vi "Test.vi"() -> ()   [LabVIEW 2017]
uses:
  <userlib>/_NEVSTOP/JKI State Machine ++/_Support/_JKISMQFGV.vi
  <userlib>/_NEVSTOP/JKI State Machine ++/JKI-State-Machine-Plus.lvlib
panel:
  out "State History":string
  in  "Name(\"\" to use uuid)":string="Event JKISM"
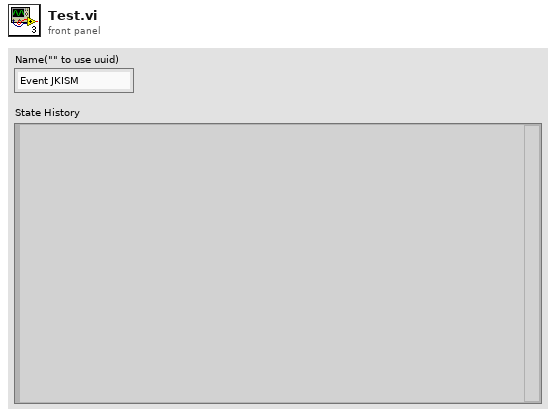
[diagram p1: front panel]
types:
  T1 = enum32{"Invalid", "Standard", "Closed", "Hidden", "Minimized", "Maximized"}
  T2 = enum32{"invalid app kind", "Development System", "Run Time System", "Student Edition", "Embedded LabVIEW", "Evaluation", "Custom"}
  T3 = cluster{"Core":cluster{"Current VI Reference":refnum<vi>, "Close Panel on Exit?":bool}, "Your Boolean data":bool, "Your string data":string}
  T4 = cluster{"Current VI Reference":refnum<vi>, "Close Panel on Exit?":bool}
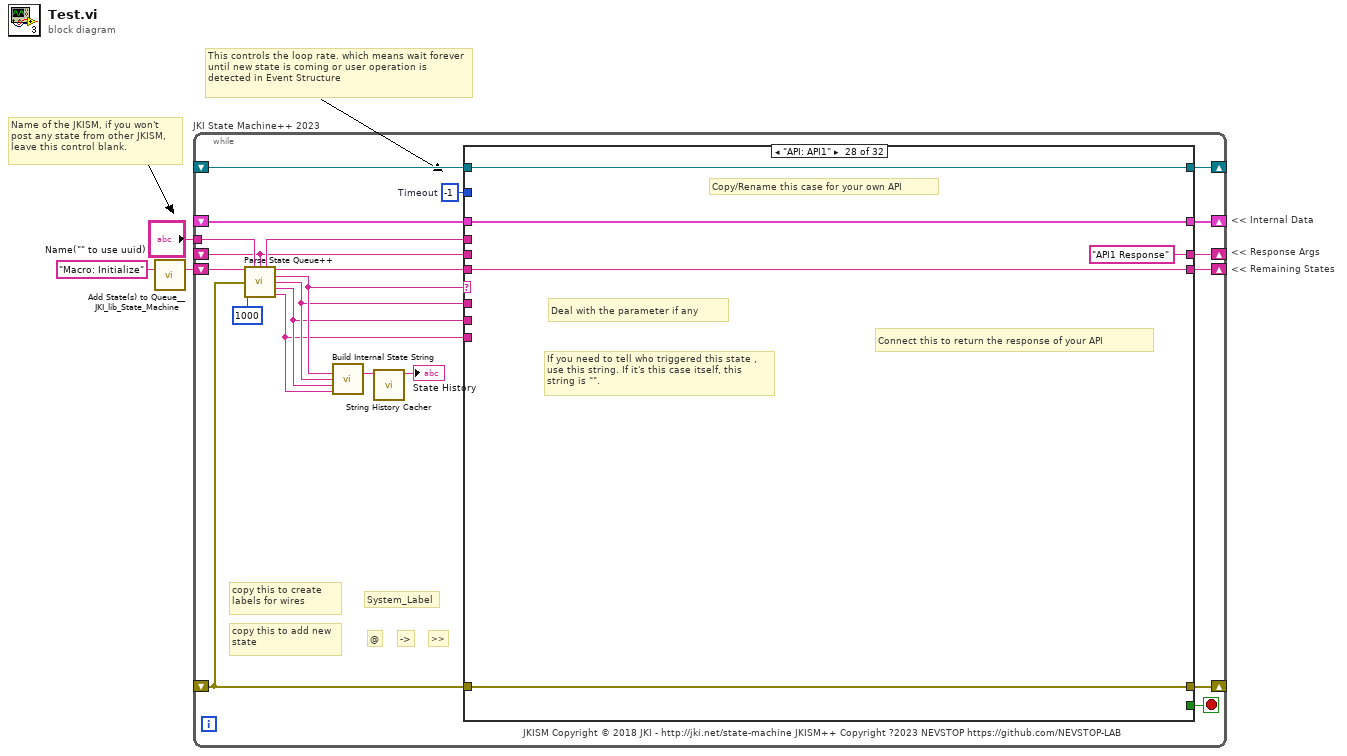
[diagram p0: block diagram]
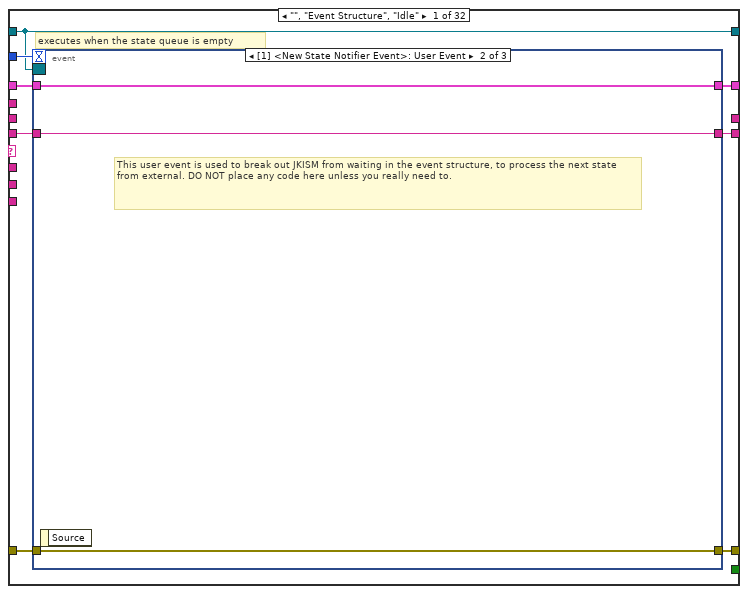
[diagram p2: hidden frame]
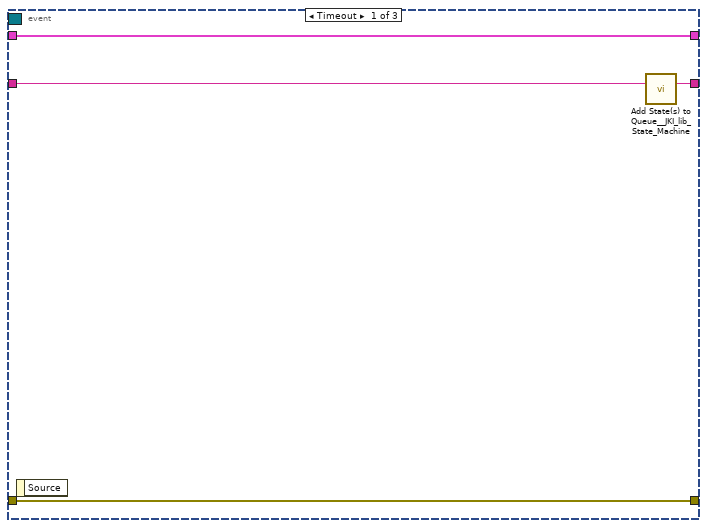
[diagram p3: hidden frame]
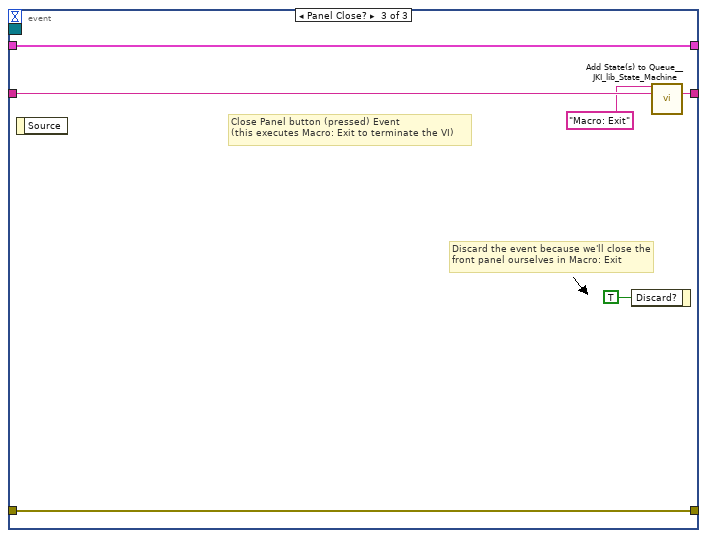
[diagram p4: hidden frame]
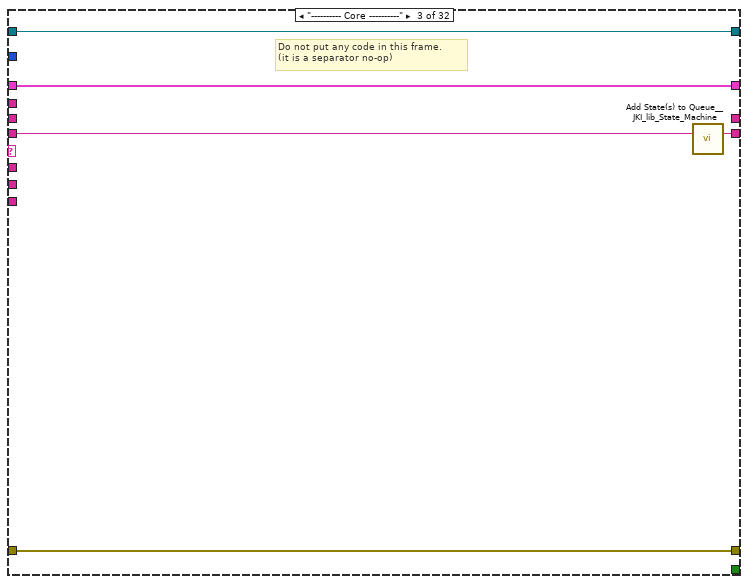
[diagram p6: hidden frame]
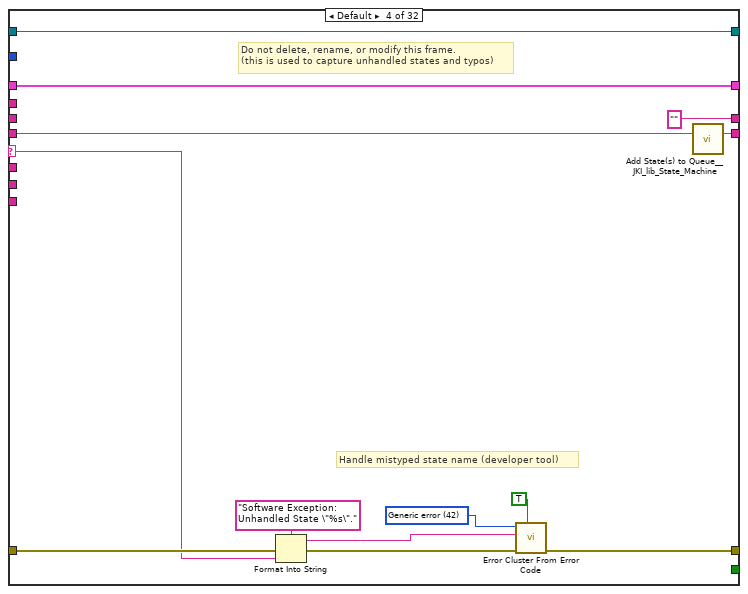
[diagram p7: hidden frame]
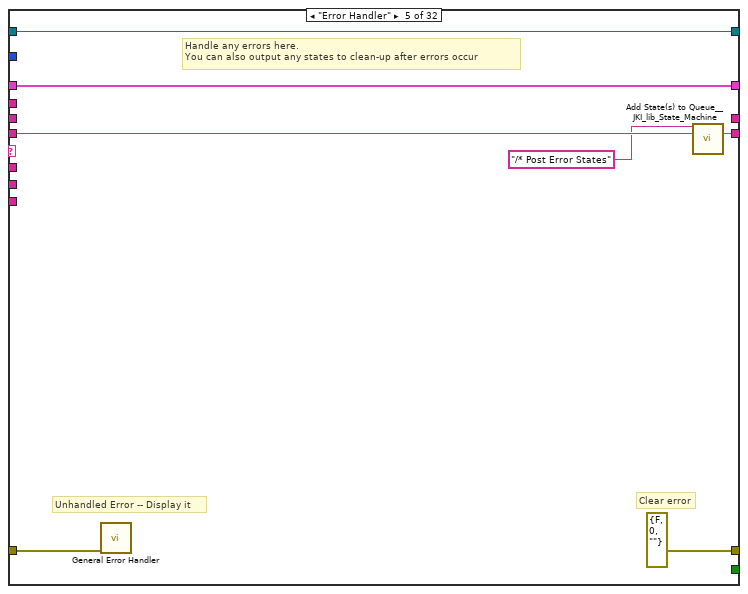
[diagram p8: hidden frame]
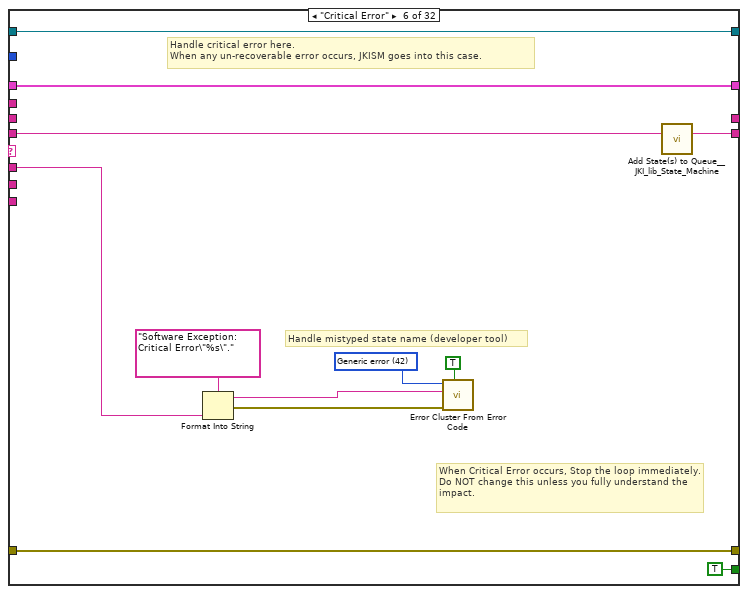
[diagram p9: hidden frame]
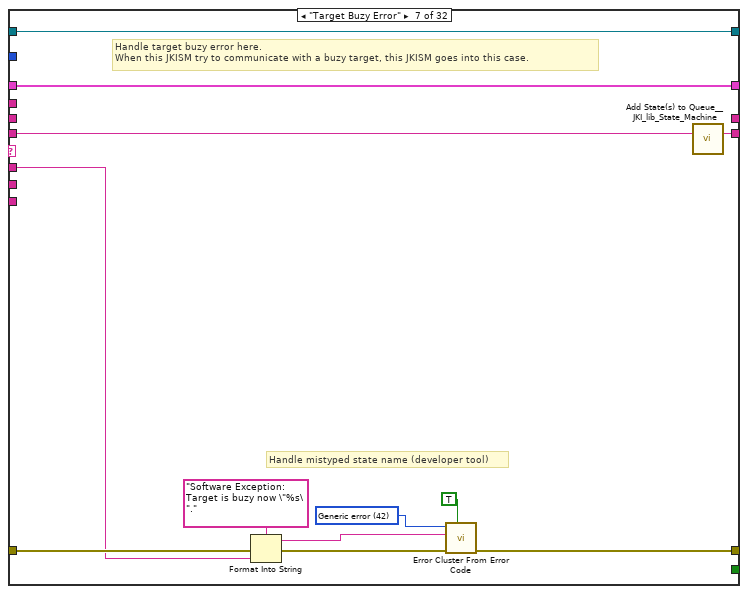
[diagram p10: hidden frame]
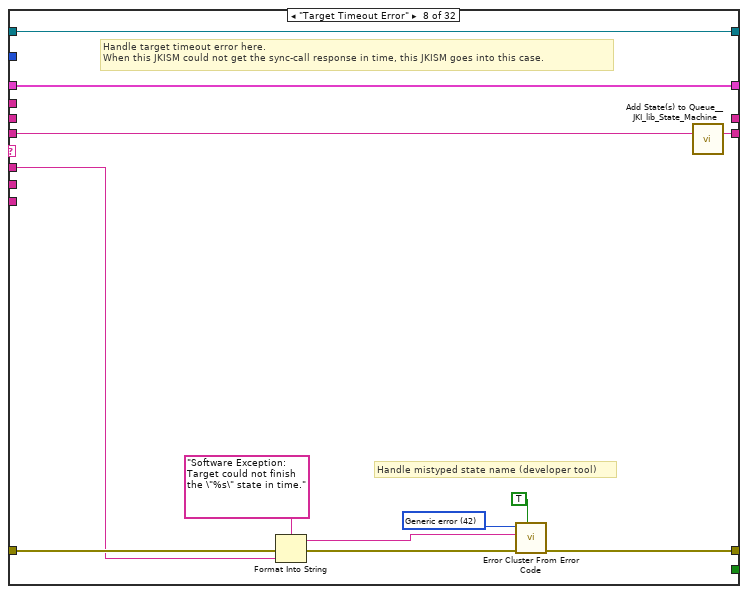
[diagram p11: hidden frame]
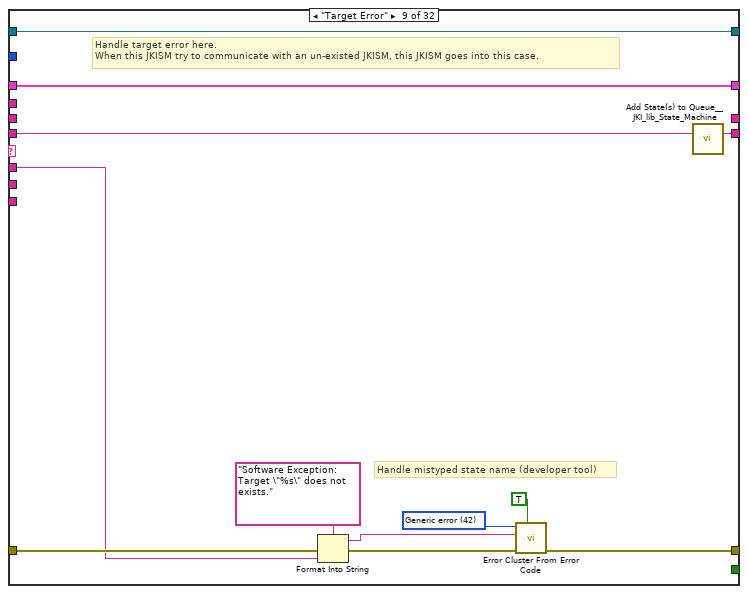
[diagram p12: hidden frame]
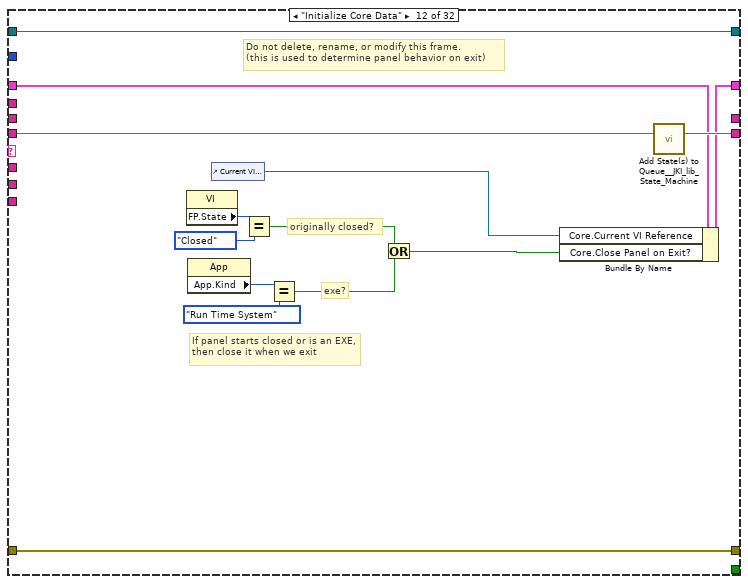
[diagram p15: hidden frame]
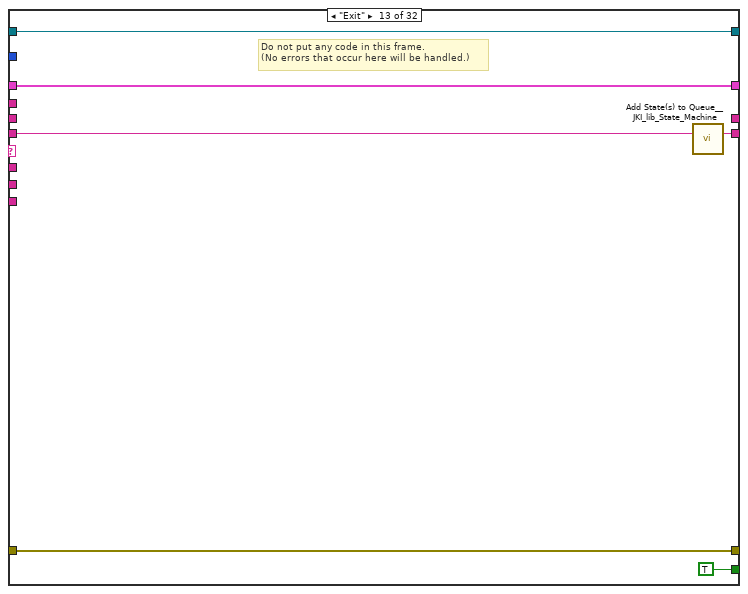
[diagram p16: hidden frame]
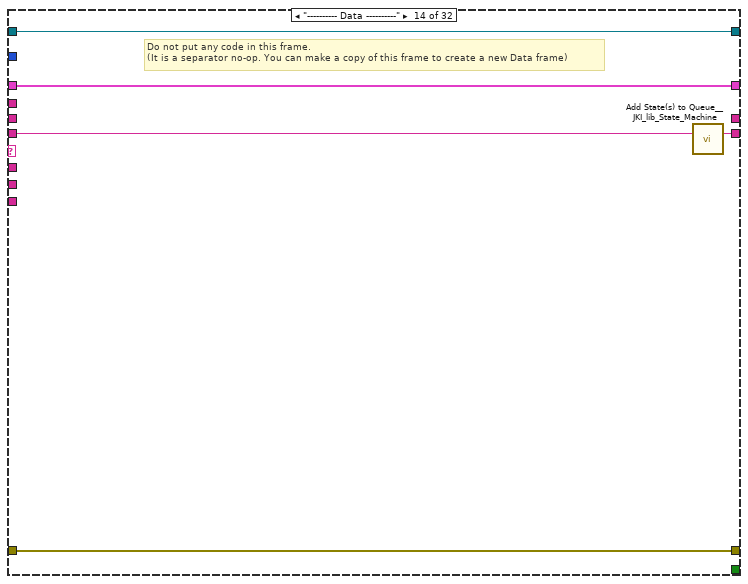
[diagram p17: hidden frame]
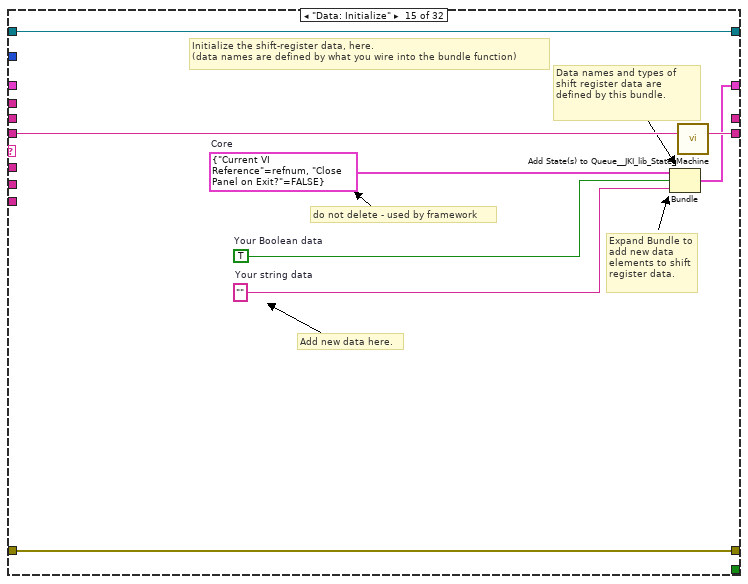
[diagram p18: hidden frame]
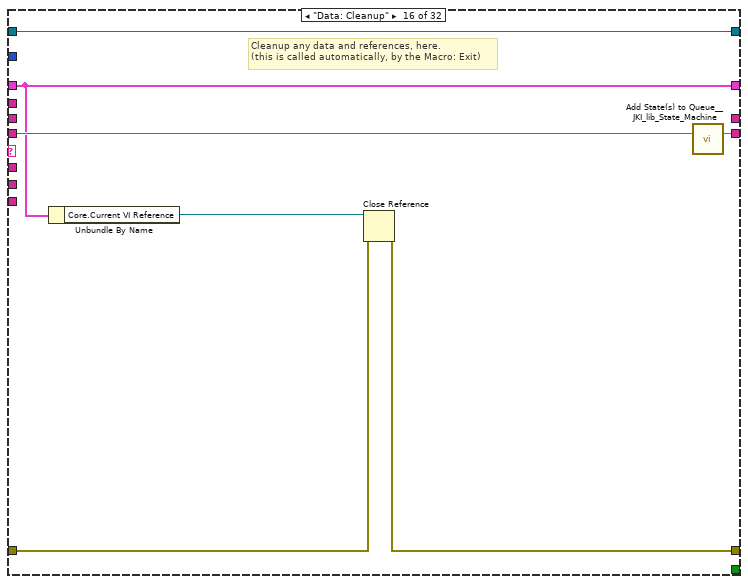
[diagram p19: hidden frame]
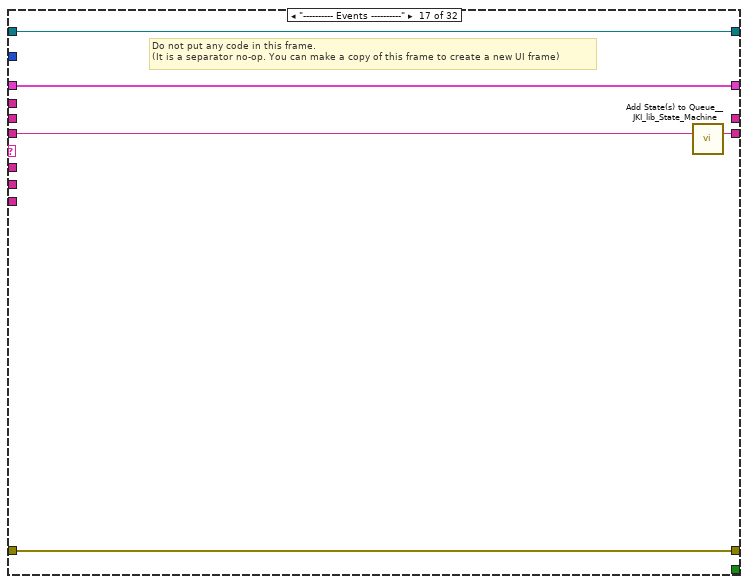
[diagram p20: hidden frame]
diagram:
  # "<< Internal Data"
  # "<< Response Args"
  # "<< Remaining States"
  # "Name of the JKISM, if you won't post any state from other JKISM,  leave this control blank."
  # "This controls the loop rate. which means wait forever until new state is coming or user operation is detected in Event Structure"
  n1 = call <vilib>:"Add State(s) to Queue__JKI_lib_State_Machine.vi"("State(s) in (\"\")"="Macro: Initialize") -> ("States Out"=w1:string)  [unwired: 14 in]
  n2 = while "JKI State Machine++ 2023" {
    shift-right: [w20] -> _
    shift-left: _ -> [w19]
    shift-right: [w23] -> _
    shift-left: _ -> [w17]
    shift-right: [w22] -> _
    shift-left: w1 -> [w24]
    tunnel: "Name(\"\" to use uuid)" -> [w12]
    shift-right: [w15] -> _
    shift-left: _ -> [w4]
    shift-right: [w14] -> _
    shift-left: _ -> [w13]
    stop <- w21 stop-if-true
    w18 = -1  # Timeout
    # "JKISM Copyright © 2018 JKI - http://jki.net/state-machine JKISM++ Copyright ?2023 NEVSTOP https://github.com/NEVSTOP-LAB"
    # "copy this to add new state"
    # ">>"
    # "->"
    # "@"
    # "copy this to create labels for wires"
    # "System_Label"
    n3 = call <userlib>:"Parse State Queue++.vi"("State Queue"=w24, "Name(\"\" to use uuid)"=w12, "Response Arguments"=w4, "Error In (no error)"=w17, "Response Timeout(5000ms)"=1000 ("Response Timeout(1000ms)")) -> ("Name Used"=w5:string, "Remaining States"=w25:string, "Current State"=w9:string, "Arguments"=w8:string, "Argument - State"=w7:string, "From Who"=w6:string)  [unwired: 5 in]
    n4 = call <userlib>:"Build Internal State String.vi"("State"=w9, "Arguments (\"\")"=w8, "Arg-State (\"\")"=w7, "Source (\"\")"=w6) -> ("State with Arguments"=w10:string)  [unwired: 11 in]
    n5 = call <userlib>:"String History Cacher.vi"("String"=w10) -> ("String Cache"=→"State History":string)  [unwired: 10 in]
    n6 = case shown="\"API: API1\"" w9 {
      selector: w9 -> [_ _ _ w58 _ _ _ _ _ _ _ _ _ _ _ _ _ _ _ _ _ _ _ _ _ _ _ _ _ _ _ _]
      tunnel: w25 -> [w33 w49 w55 w62 w75 w85 w88 w105 w117 w126 w130 w145 w151 w156 w164 w171 w176 w182 w186 w192 w197 w204 w216 w286 w292 w303 w306 w311 w317 w325 w331 w337]
      tunnel: w8 -> [_ _ _ _ _ w78 w90 w101 w113 _ _ _ _ _ _ _ _ _ _ _ _ w199 w210 _ _ _ _ _ w314 _ _ _]
      tunnel: w19 -> [w31 w48 w52 w60 w72 w86 w92 w103 w115 w125 w129 w138 w149 w153 _ w166 w173 w181 w185 w189 w195 w202 w212 w283 w289 w300 w305 w310 w316 w322 w328 w334]
      tunnel: [w30 w50 w53 w64 errorcluster {"status"=FALSE, "code"=0, "source"=""} ("error out") w87 w95 w107 w119 w127 w131 w142 w148 w154 w161 w167 w174 w177 w184 w190 w194 w200 w213 w284 w290 w301 w307 w312 w318 w323 w329 w335] -> w23
      tunnel: w17 -> [w29 w50 w53 w63 w71 w87 w94 w106 w118 w127 w131 w142 w148 w154 w161 w168 w174 _ w187 w190 w194 w201 w214 w284 w290 w301 w307 w312 w318 w323 w329 w335]
      tunnel: [w32 w49 w54 w61 w74 w84 w93 w104 w116 w126 w130 w144 w150 w155 w163 w170 w175 w182 w186 w191 w196 w203 w215 w285 w291 w302 w306 w311 w317 w324 w330 w336] -> w22
      tunnel: [_ _ _ _ _ TRUE _ _ _ _ _ _ TRUE _ _ _ _ _ _ _ _ _ _ _ _ _ _ _ _ _ _ _] -> w21
      tunnel: [w28 w48 w52 w60 w72 w86 w92 w103 w115 w125 w129 w143 w149 w153 w162 w166 w173 w181 w185 w189 w195 w202 w212 w283 w289 w300 w305 w310 w316 w322 w328 w334] -> w20
      tunnel: w18 -> [w27 _ _ _ _ _ _ _ _ _ _ _ _ _ _ _ _ _ _ _ _ _ _ _ _ _ _ _ _ _ _ _]
      tunnel: w6 -> [_ _ _ _ _ _ _ _ _ _ _ _ _ _ _ _ _ _ _ _ _ _ _ _ _ _ _ _ _ _ _ _]
      tunnel: w7 -> [_ _ _ _ _ _ _ _ _ _ _ _ _ _ _ _ _ _ _ _ _ _ _ _ _ _ _ _ _ _ _ _]
      tunnel: [_ _ _ "" _ _ _ _ _ _ _ _ _ _ _ _ _ _ _ _ _ _ _ _ _ _ _ "API1 Response" w313 _ "DoA Finished" "DoB Finished"] -> w15
      tunnel: [w26 w47 w51 w56 w69 w76 w89 w100 w112 w124 w128 w132 w146 w152 w157 w165 w172 w180 w183 w188 w193 w198 w209 w282 w287 w293 w304 w309 w315 w321 w327 w333] -> w14
      tunnel: w13 -> [w26 w47 w51 w56 w69 w76 w89 w100 w112 w124 w128 w132 w146 w152 w157 w165 w172 _ w183 w188 w193 w198 w209 w282 w287 w293 w304 w309 w315 w321 w327 w333]
      tunnel: w5 -> [_ _ _ _ _ _ _ _ _ _ _ _ _ _ _ _ _ w179 _ _ _ _ _ _ _ _ _ _ _ _ _ _]
      tunnel: w4 -> [_ _ _ _ _ _ _ _ _ _ _ _ _ _ _ _ _ _ _ _ _ _ _ _ _ _ _ _ _ _ _ _]
      frame "", "Event Structure", "Idle" {
        # "executes when the state queue is empty"
        n7 = event shown="[1] <New State Notifier Event>: User Event" {
          selector: w26 -> [_ _ _]
          dyn-events: _ -> [_ _ _]
          timeout: w27 -> [_ _ _]
          tunnel: w33 -> [w37 w39 w46]
          tunnel: [w36 w39 w45] -> w32
          tunnel: w31 -> [w34 w40 w43]
          tunnel: [w35 w38 w44] -> w30
          tunnel: w29 -> [w35 w38 w44]
          tunnel: [w34 w40 w43] -> w28
          event Timeout {
            n8 = event-data() -> ()  [unwired: 1 in, 1 out]
            n9 = call <vilib>:"Add State(s) to Queue__JKI_lib_State_Machine.vi"("State(s) in (\"\")"=w37) -> ("States Out"=w36:string)  [unwired: 14 in]
          }
          event User Event {
            # "This user event is used to break out JKISM from waiting in the event structure, to process the next state from external. DO NOT place any code here unless you really need to."
            n10 = event-data() -> ()  [unwired: 1 in, 1 out]
          }
          event Panel Close? {
            # "Discard the event because we'll close the front panel ourselves in Macro: Exit"
            # "Close Panel button (pressed) Event\n(this executes Macro: Exit to terminate the VI)"
            n11 = event-data() -> ()  [unwired: 1 in, 1 out]
            n12 = event-data("Discard?"=TRUE) -> ()  [unwired: 1 in, 1 out]
            n13 = call <vilib>:"Add State(s) to Queue__JKI_lib_State_Machine.vi"("State(s) in Front (\"\")"="Macro: Exit", "State(s) in (\"\")"=w46) -> ("States Out"=w45:string)  [unwired: 13 in]
          }
        }
      }
      frame "JKISM++ Documentation" {
        # "JKISM++ Documentation"
        # "State Syntax:\nStateCategory: State >> Argument @|-> JKISMName\nLine Terminator: Line feed\n\nExample:\nUI: Help >> About @Main\nUI: Help >> About ->Main"
        # "Commenting:\nTo add a comment use \"//\" or \"#\" and all text to the right will be ignored\nCommenting Example:\nUI: Initialize // This initializes the UI\n# This whole line is a comment\n// Another comment line"
        # "Where \"UI\" is the state category\nWhere \"Help\" is the state\nWhere \"About\" is the argument\nWhere \"Main\" is the Name of JKISM,which actually run the \"UI: Help >> About\"\n\n    \"@\" stands for sync state. Current JKISM will wait until the state is finished. \n            - if \"Main\" named JKISM does not exist, \"Target Error\" will occur.\n            - if \"Main\" named JKISM is in another sync remote state, \"Target Buzy Error\" will occur.\n            - if \"Main\" named JKISM could not finish the state in time, \"Target Timeout Error\" will occur.\n            - if everything is right. \"Response\" will occur with Argument back from \"Main\" named JKISM. \n\n    \"->\" stands for async state. Current JKISM will post the state and continue to next state in next iteration.\n            - if \"Main\" named JKISM does not exist, \"Target Error\" will occur.\n            - if everything is right. \"Async Message Posted\" will occur.\n            - After State is finished. Caller will receive a \"Async Response\" state from callee.\n\nWhen duplicated name is used for multiple JKISM module or some framework problem happens, \"Critical Error\" will occur."
      }
      frame "---------- Core ----------" {
        # "Do not put any code in this frame.\n(it is a separator no-op)"
        n14 = call <vilib>:"Add State(s) to Queue__JKI_lib_State_Machine.vi"("State(s) in (\"\")"=w55) -> ("States Out"=w54:string)  [unwired: 14 in]
      }
      frame Default {
        w67 = 42 items=["No error", "Argument error", "Memory is full", "Out of zone", "End of file", "File already open", "Generic file I/O error", "File not found", "File permission error", "Disk is full", "Duplicate path", "Too many files open", "System feature not enabled", "Resource file not found", "Cannot add resource", "Resource not found", "Image not found", "Image memory error", "Pen does not exist", "Config type invalid", "Config token not found", "Config parse error", "Config memory error", "Bad external code format", "Bad external code offset", "External code not present", "Null window", "Destroy window error", "Null menu", "Print aborted", "Bad print record", "Print driver error", "Windows error during printing", "Memory error during printing", "Print dialog error", "Generic print error", "Invalid device refnum", "Device not found", "Device parameter error", "Device unit error", "Cannot open device", "Device call aborted", "Generic error", "Cancelled by user", "Object ID too low", "Object ID too high", "Object not in heap", "Unknown heap", "Unknown object (invalid DefProc)", "Unknown object (DefProc not in table)", "Message out of range", "Invalid (null) method", "Unknown message", "Manager call not supported", "Bad address", "Network operation in progress", "Network operation timed out", "Connection is busy", "Network attribute not supported", "Network error", "Address in use", "System out of memory", "Connection aborted", "Connection refused", "Not connected", "Already connected", "Connection closed", "Initialization error (interapplication manager)", "Bad occurrence", "Wait on unbound occurrence handler", "Occurrence queue overflow", "Datalog type conflict", "Unused", "Unrecognized type (interapplication manager)", "Memory corrupt", "Failed to make temporary DLL", "Old CIN version", "Drag socket not found", "Failed to load drop-object", "Failed to register OLE object", "Failed to release OLE object", "Format specifier type mismatch", "Unknown format specifier", "Too few format specifiers", "Too many format specifiers", "Scan failed", "Newer CIN version", "Error converting to variant", "Runtime menu error", "Password tampered", "Variant attribute not found", "Incompatible variant data type", "Event data is not available", "Event Store is not present", "Occurrence is not found", "Event Queue is not created", "Event info is not available", "Refnum passed is NULL", "Error retrieving Class GUID", "Error retrieving CoClass GUID", "Error retrieving TypeLib GUID.", "Bad built application magic bytes.", "Specific driver is different from the specific driver associated with the Logical Name.", "There is no session opened to the class driver.", "Max Error", "MAX - Error with config objects", "MAX - Error loading configuration", "MAX - Group not supported"]
        # "Do not delete, rename, or modify this frame.\n(this is used to capture unhandled states and typos)"
        # "Handle mistyped state name (developer tool)"
        n15 = Format Into String(format string="Software Exception: Unhandled State \"%s\"." ("message"), error in=w63, w58) -> (resulting string=w66:string, error out=w65:errorcluster)  [unwired: 1 in]
        n16 = call <vilib>:"Error Cluster From Error Code.vi"("show call chain? (False)"=TRUE, "error in (no error)"=w65, "error message (\"\")"=w66, "error code (0)"=w67) -> ("error out"=w64:errorcluster)  [unwired: 5 in]
        n17 = call <vilib>:"Add State(s) to Queue__JKI_lib_State_Machine.vi"("State(s) in (\"\")"=w62) -> ("States Out"=w61:string)  [unwired: 14 in]
      }
      frame "Error Handler" {
        # "Unhandled Error -- Display it"
        # "Handle any errors here.\nYou can also output any states to clean-up after errors occur"
        # "Clear error"
        n18 = call <vilib>:"General Error Handler.vi"("error in (no error)"=w71) -> ()  [unwired: 10 in, 5 out]
        n19 = call <vilib>:"Add State(s) to Queue__JKI_lib_State_Machine.vi"("State(s) in Front (\"\")"="/* Post Error States", "State(s) in (\"\")"=w75) -> ("States Out"=w74:string)  [unwired: 13 in]
      }
      frame "Critical Error" {
        w82 = 42 items=["No error", "Argument error", "Memory is full", "Out of zone", "End of file", "File already open", "Generic file I/O error", "File not found", "File permission error", "Disk is full", "Duplicate path", "Too many files open", "System feature not enabled", "Resource file not found", "Cannot add resource", "Resource not found", "Image not found", "Image memory error", "Pen does not exist", "Config type invalid", "Config token not found", "Config parse error", "Config memory error", "Bad external code format", "Bad external code offset", "External code not present", "Null window", "Destroy window error", "Null menu", "Print aborted", "Bad print record", "Print driver error", "Windows error during printing", "Memory error during printing", "Print dialog error", "Generic print error", "Invalid device refnum", "Device not found", "Device parameter error", "Device unit error", "Cannot open device", "Device call aborted", "Generic error", "Cancelled by user", "Object ID too low", "Object ID too high", "Object not in heap", "Unknown heap", "Unknown object (invalid DefProc)", "Unknown object (DefProc not in table)", "Message out of range", "Invalid (null) method", "Unknown message", "Manager call not supported", "Bad address", "Network operation in progress", "Network operation timed out", "Connection is busy", "Network attribute not supported", "Network error", "Address in use", "System out of memory", "Connection aborted", "Connection refused", "Not connected", "Already connected", "Connection closed", "Initialization error (interapplication manager)", "Bad occurrence", "Wait on unbound occurrence handler", "Occurrence queue overflow", "Datalog type conflict", "Unused", "Unrecognized type (interapplication manager)", "Memory corrupt", "Failed to make temporary DLL", "Old CIN version", "Drag socket not found", "Failed to load drop-object", "Failed to register OLE object", "Failed to release OLE object", "Format specifier type mismatch", "Unknown format specifier", "Too few format specifiers", "Too many format specifiers", "Scan failed", "Newer CIN version", "Error converting to variant", "Runtime menu error", "Password tampered", "Variant attribute not found", "Incompatible variant data type", "Event data is not available", "Event Store is not present", "Occurrence is not found", "Event Queue is not created", "Event info is not available", "Refnum passed is NULL", "Error retrieving Class GUID", "Error retrieving CoClass GUID", "Error retrieving TypeLib GUID.", "Bad built application magic bytes.", "Specific driver is different from the specific driver associated with the Logical Name.", "There is no session opened to the class driver.", "Max Error", "MAX - Error with config objects", "MAX - Error loading configuration", "MAX - Group not supported"]
        # "Handle critical error here.\nWhen any un-recoverable error occurs, JKISM goes into this case."
        # "When Critical Error occurs, Stop the loop immediately. Do NOT change this unless you fully understand the impact."
        # "Handle mistyped state name (developer tool)"
        n20 = Format Into String(format string="Software Exception: Critical Error\"%s\"." ("message"), w78) -> (resulting string=w81:string, error out=w80:errorcluster)  [unwired: 2 in]
        n21 = call <vilib>:"Error Cluster From Error Code.vi"("show call chain? (False)"=TRUE, "error in (no error)"=w80, "error message (\"\")"=w81, "error code (0)"=w82) -> ()  [unwired: 5 in, 1 out]
        n22 = call <vilib>:"Add State(s) to Queue__JKI_lib_State_Machine.vi"("State(s) in (\"\")"=w85) -> ("States Out"=w84:string)  [unwired: 14 in]
      }
      frame "Target Buzy Error" {
        w98 = 42 items=["No error", "Argument error", "Memory is full", "Out of zone", "End of file", "File already open", "Generic file I/O error", "File not found", "File permission error", "Disk is full", "Duplicate path", "Too many files open", "System feature not enabled", "Resource file not found", "Cannot add resource", "Resource not found", "Image not found", "Image memory error", "Pen does not exist", "Config type invalid", "Config token not found", "Config parse error", "Config memory error", "Bad external code format", "Bad external code offset", "External code not present", "Null window", "Destroy window error", "Null menu", "Print aborted", "Bad print record", "Print driver error", "Windows error during printing", "Memory error during printing", "Print dialog error", "Generic print error", "Invalid device refnum", "Device not found", "Device parameter error", "Device unit error", "Cannot open device", "Device call aborted", "Generic error", "Cancelled by user", "Object ID too low", "Object ID too high", "Object not in heap", "Unknown heap", "Unknown object (invalid DefProc)", "Unknown object (DefProc not in table)", "Message out of range", "Invalid (null) method", "Unknown message", "Manager call not supported", "Bad address", "Network operation in progress", "Network operation timed out", "Connection is busy", "Network attribute not supported", "Network error", "Address in use", "System out of memory", "Connection aborted", "Connection refused", "Not connected", "Already connected", "Connection closed", "Initialization error (interapplication manager)", "Bad occurrence", "Wait on unbound occurrence handler", "Occurrence queue overflow", "Datalog type conflict", "Unused", "Unrecognized type (interapplication manager)", "Memory corrupt", "Failed to make temporary DLL", "Old CIN version", "Drag socket not found", "Failed to load drop-object", "Failed to register OLE object", "Failed to release OLE object", "Format specifier type mismatch", "Unknown format specifier", "Too few format specifiers", "Too many format specifiers", "Scan failed", "Newer CIN version", "Error converting to variant", "Runtime menu error", "Password tampered", "Variant attribute not found", "Incompatible variant data type", "Event data is not available", "Event Store is not present", "Occurrence is not found", "Event Queue is not created", "Event info is not available", "Refnum passed is NULL", "Error retrieving Class GUID", "Error retrieving CoClass GUID", "Error retrieving TypeLib GUID.", "Bad built application magic bytes.", "Specific driver is different from the specific driver associated with the Logical Name.", "There is no session opened to the class driver.", "Max Error", "MAX - Error with config objects", "MAX - Error loading configuration", "MAX - Group not supported"]
        # "Handle target buzy error here.\nWhen this JKISM try to communicate with a buzy target, this JKISM goes into this case."
        # "Handle mistyped state name (developer tool)"
        n23 = Format Into String(format string="Software Exception: Target is buzy now \"%s\"." ("message"), error in=w94, w90) -> (resulting string=w97:string, error out=w96:errorcluster)  [unwired: 1 in]
        n24 = call <vilib>:"Error Cluster From Error Code.vi"("show call chain? (False)"=TRUE, "error in (no error)"=w96, "error message (\"\")"=w97, "error code (0)"=w98) -> ("error out"=w95:errorcluster)  [unwired: 5 in]
        n25 = call <vilib>:"Add State(s) to Queue__JKI_lib_State_Machine.vi"("State(s) in (\"\")"=w88) -> ("States Out"=w93:string)  [unwired: 14 in]
      }
      frame "Target Timeout Error" {
        w110 = 42 items=["No error", "Argument error", "Memory is full", "Out of zone", "End of file", "File already open", "Generic file I/O error", "File not found", "File permission error", "Disk is full", "Duplicate path", "Too many files open", "System feature not enabled", "Resource file not found", "Cannot add resource", "Resource not found", "Image not found", "Image memory error", "Pen does not exist", "Config type invalid", "Config token not found", "Config parse error", "Config memory error", "Bad external code format", "Bad external code offset", "External code not present", "Null window", "Destroy window error", "Null menu", "Print aborted", "Bad print record", "Print driver error", "Windows error during printing", "Memory error during printing", "Print dialog error", "Generic print error", "Invalid device refnum", "Device not found", "Device parameter error", "Device unit error", "Cannot open device", "Device call aborted", "Generic error", "Cancelled by user", "Object ID too low", "Object ID too high", "Object not in heap", "Unknown heap", "Unknown object (invalid DefProc)", "Unknown object (DefProc not in table)", "Message out of range", "Invalid (null) method", "Unknown message", "Manager call not supported", "Bad address", "Network operation in progress", "Network operation timed out", "Connection is busy", "Network attribute not supported", "Network error", "Address in use", "System out of memory", "Connection aborted", "Connection refused", "Not connected", "Already connected", "Connection closed", "Initialization error (interapplication manager)", "Bad occurrence", "Wait on unbound occurrence handler", "Occurrence queue overflow", "Datalog type conflict", "Unused", "Unrecognized type (interapplication manager)", "Memory corrupt", "Failed to make temporary DLL", "Old CIN version", "Drag socket not found", "Failed to load drop-object", "Failed to register OLE object", "Failed to release OLE object", "Format specifier type mismatch", "Unknown format specifier", "Too few format specifiers", "Too many format specifiers", "Scan failed", "Newer CIN version", "Error converting to variant", "Runtime menu error", "Password tampered", "Variant attribute not found", "Incompatible variant data type", "Event data is not available", "Event Store is not present", "Occurrence is not found", "Event Queue is not created", "Event info is not available", "Refnum passed is NULL", "Error retrieving Class GUID", "Error retrieving CoClass GUID", "Error retrieving TypeLib GUID.", "Bad built application magic bytes.", "Specific driver is different from the specific driver associated with the Logical Name.", "There is no session opened to the class driver.", "Max Error", "MAX - Error with config objects", "MAX - Error loading configuration", "MAX - Group not supported"]
        # "Handle target timeout error here.\nWhen this JKISM could not get the sync-call response in time, this JKISM goes into this case."
        # "Handle mistyped state name (developer tool)"
        n26 = Format Into String(format string="Software Exception: Target could not finish the \"%s\" state in time." ("message"), error in=w106, w101) -> (resulting string=w109:string, error out=w108:errorcluster)  [unwired: 1 in]
        n27 = call <vilib>:"Error Cluster From Error Code.vi"("show call chain? (False)"=TRUE, "error in (no error)"=w108, "error message (\"\")"=w109, "error code (0)"=w110) -> ("error out"=w107:errorcluster)  [unwired: 5 in]
        n28 = call <vilib>:"Add State(s) to Queue__JKI_lib_State_Machine.vi"("State(s) in (\"\")"=w105) -> ("States Out"=w104:string)  [unwired: 14 in]
      }
      frame "Target Error" {
        w122 = 42 items=["No error", "Argument error", "Memory is full", "Out of zone", "End of file", "File already open", "Generic file I/O error", "File not found", "File permission error", "Disk is full", "Duplicate path", "Too many files open", "System feature not enabled", "Resource file not found", "Cannot add resource", "Resource not found", "Image not found", "Image memory error", "Pen does not exist", "Config type invalid", "Config token not found", "Config parse error", "Config memory error", "Bad external code format", "Bad external code offset", "External code not present", "Null window", "Destroy window error", "Null menu", "Print aborted", "Bad print record", "Print driver error", "Windows error during printing", "Memory error during printing", "Print dialog error", "Generic print error", "Invalid device refnum", "Device not found", "Device parameter error", "Device unit error", "Cannot open device", "Device call aborted", "Generic error", "Cancelled by user", "Object ID too low", "Object ID too high", "Object not in heap", "Unknown heap", "Unknown object (invalid DefProc)", "Unknown object (DefProc not in table)", "Message out of range", "Invalid (null) method", "Unknown message", "Manager call not supported", "Bad address", "Network operation in progress", "Network operation timed out", "Connection is busy", "Network attribute not supported", "Network error", "Address in use", "System out of memory", "Connection aborted", "Connection refused", "Not connected", "Already connected", "Connection closed", "Initialization error (interapplication manager)", "Bad occurrence", "Wait on unbound occurrence handler", "Occurrence queue overflow", "Datalog type conflict", "Unused", "Unrecognized type (interapplication manager)", "Memory corrupt", "Failed to make temporary DLL", "Old CIN version", "Drag socket not found", "Failed to load drop-object", "Failed to register OLE object", "Failed to release OLE object", "Format specifier type mismatch", "Unknown format specifier", "Too few format specifiers", "Too many format specifiers", "Scan failed", "Newer CIN version", "Error converting to variant", "Runtime menu error", "Password tampered", "Variant attribute not found", "Incompatible variant data type", "Event data is not available", "Event Store is not present", "Occurrence is not found", "Event Queue is not created", "Event info is not available", "Refnum passed is NULL", "Error retrieving Class GUID", "Error retrieving CoClass GUID", "Error retrieving TypeLib GUID.", "Bad built application magic bytes.", "Specific driver is different from the specific driver associated with the Logical Name.", "There is no session opened to the class driver.", "Max Error", "MAX - Error with config objects", "MAX - Error loading configuration", "MAX - Group not supported"]
        # "Handle target error here.\nWhen this JKISM try to communicate with an un-existed JKISM, this JKISM goes into this case."
        # "Handle mistyped state name (developer tool)"
        n29 = Format Into String(format string="Software Exception: Target \"%s\" does not exists." ("message"), error in=w118, w113) -> (resulting string=w121:string, error out=w120:errorcluster)  [unwired: 1 in]
        n30 = call <vilib>:"Error Cluster From Error Code.vi"("show call chain? (False)"=TRUE, "error in (no error)"=w120, "error message (\"\")"=w121, "error code (0)"=w122) -> ("error out"=w119:errorcluster)  [unwired: 5 in]
        n31 = call <vilib>:"Add State(s) to Queue__JKI_lib_State_Machine.vi"("State(s) in (\"\")"=w117) -> ("States Out"=w116:string)  [unwired: 14 in]
      }
      frame "Async Response", "Response" {
        # "Handle Async-call Response (\"Async Response\" for ->)"
        # "Handle Sync-call Response (\"Response\" for @)"
        # "After Message is excuted, JKISM+ goes to this state for recieve the response. \n    For Async Message(->), \"Async Response\" is used. This JKISM will goes to \"Async Message Posted\" immediately and recieve the \"Async Response\" after the callee finishes the message.\n    For Sync Message(@),  This JKISM will wait until the message is done and immidieatly goes to \"Response\""
      }
      frame "Async Message Posted" {
        # "Handle post action for async message (->)."
        # "After Async Message is posted (->), JKISM+ goes to this state for post-action. You can use Argument - State to tell which Async Message is called."
      }
      frame "Initialize Core Data" {
        # "Do not delete, rename, or modify this frame.\n(this is used to determine panel behavior on exit)"
        # "originally closed?"
        # "exe?"
        # "If panel starts closed or is an EXE, then close it when we exit"
        n32 = property class="VI"() -> ("FP.State"=w135:T1)  [unwired: 2 in, 2 out]
        n33 = property class="App"() -> ("App.Kind"=w141:T2)  [unwired: 2 in, 2 out]
        n34 = control-ref of="Current VI Reference"() -> (w136:refnum<vi>)
        n35 = Equal?(x=w135, y=T1."Closed" ("Front Panel Window:State")) -> (x = y?=w133:bool)
        n36 = Equal?(x=w141, y=T2."Run Time System" ("Application:Kind")) -> (x = y?=w139:bool)
        n37 = Or(x=w133, y=w139) -> (x .or. y?=w137:bool)
        n38 = Bundle By Name(cluster=w138, "Core.Current VI Reference"=w136, "Core.Close Panel on Exit?"=w137) -> (w143:T3)
        n39 = call <vilib>:"Add State(s) to Queue__JKI_lib_State_Machine.vi"("State(s) in (\"\")"=w145) -> ("States Out"=w144:string)  [unwired: 14 in]
      }
      frame "Exit" {
        # "Do not put any code in this frame.\n(No errors that occur here will be handled.)"
        n40 = call <vilib>:"Add State(s) to Queue__JKI_lib_State_Machine.vi"("State(s) in (\"\")"=w151) -> ("States Out"=w150:string)  [unwired: 14 in]
      }
      frame "---------- Data ----------" {
        # "Do not put any code in this frame.\n(It is a separator no-op. You can make a copy of this frame to create a new Data frame)"
        n41 = call <vilib>:"Add State(s) to Queue__JKI_lib_State_Machine.vi"("State(s) in (\"\")"=w156) -> ("States Out"=w155:string)  [unwired: 14 in]
      }
      frame "Data: Initialize" {
        w158 = T4 {"Current VI Reference"=refnum, "Close Panel on Exit?"=FALSE}  # Core
        w160 = TRUE  # Your Boolean data
        w159 = ""  # Your string data
        # "do not delete - used by framework"
        # "Expand Bundle to add new data elements to shift register data."
        # "Add new data here."
        # "Data names and types of shift register data are defined by this bundle."
        # "Initialize the shift-register data, here.\n(data names are defined by what you wire into the bundle function)"
        n42 = Bundle("Core"=w158, "Your Boolean data"=w160, "Your string data"=w159) -> (w162:T3)  [unwired: 1 in]
        n43 = call <vilib>:"Add State(s) to Queue__JKI_lib_State_Machine.vi"("State(s) in (\"\")"=w164) -> ("States Out"=w163:string)  [unwired: 14 in]
      }
      frame "Data: Cleanup" {
        # "Cleanup any data and references, here.\n(this is called automatically, by the Macro: Exit)"
        n44 = Unbundle By Name(w166) -> ("Core.Current VI Reference"=w169:refnum<vi>)
        n45 = Close Reference(reference=w169, error in (no error)=w168) -> (error out=w167:errorcluster)
        n46 = call <vilib>:"Add State(s) to Queue__JKI_lib_State_Machine.vi"("State(s) in (\"\")"=w171) -> ("States Out"=w170:string)  [unwired: 14 in]
      }
      frame "---------- Events ----------" {
        # "Do not put any code in this frame.\n(It is a separator no-op. You can make a copy of this frame to create a new UI frame)"
        n47 = call <vilib>:"Add State(s) to Queue__JKI_lib_State_Machine.vi"("State(s) in (\"\")"=w176) -> ("States Out"=w175:string)  [unwired: 14 in]
      }
      frame "Events: Register" {
        # "Register message event to break Waiting in Event structure."
        n48 = call <userlib>:"JKISM++ Get New State Notifier Event.vi"("Name(\"\" to use uuid) in"=w179) -> ("Error out"=w177:errorcluster, "New State Notifier Event"=w178:refnum<user-event>)  [unwired: 9 in]
        n49 = register-events(w178) -> (reference out=w180:refnum<event-registration>)  [unwired: 2 in, 1 out]
      }
      frame "Events: Unregister" {
        n50 = Unregister For Events(event registration refnum=w183, error in=w187) -> (error out=w184:errorcluster)
      }
      frame "---------- UI ----------" {
        # "Do not put any code in this frame.\n(It is a separator no-op. You can make a copy of this frame to create a new UI frame)"
        n51 = call <vilib>:"Add State(s) to Queue__JKI_lib_State_Machine.vi"("State(s) in (\"\")"=w192) -> ("States Out"=w191:string)  [unwired: 14 in]
      }
      frame "UI: Initialize" {
        # "Initialize the User Interface, here.\n(this is called automatically, by the Macro: Init)"
        n52 = call <vilib>:"Add State(s) to Queue__JKI_lib_State_Machine.vi"("State(s) in (\"\")"=w197) -> ("States Out"=w196:string)  [unwired: 14 in]
      }
      frame "UI: Cursor Set" {
        # "Argument"
        # "Set and Unset Cursor Busy.\n(Usage: \"UI: Cursor Set >> Busy|Idle\")"
        n53 = case shown="\"Idle\", Default" w199 {
          tunnel: w201 -> [w206 w208]
          tunnel: [w205 w207] -> w200
          frame "Idle", Default {
            n54 = call <vilib>:"Unset Busy.vi"("error in (no error)"=w206) -> ("error out"=w205:errorcluster)  [unwired: 10 in]
          }
          frame "Busy" {
            n55 = call <vilib>:"Set Busy.vi"("error in (no error)"=w208) -> ("error out"=w207:errorcluster)  [unwired: 9 in, 1 out]
          }
        }
        n56 = call <vilib>:"Add State(s) to Queue__JKI_lib_State_Machine.vi"("State(s) in (\"\")"=w204) -> ("States Out"=w203:string)  [unwired: 14 in]
      }
      frame "UI: Front Panel State" {
        # "Argument"
        # "Set Front Panel Open or Closed\n(Usage: \"UI: Front Panel State >> Open|Close\")"
        n57 = Unbundle By Name(w212) -> ("Core.Current VI Reference"=w211:refnum<vi>)
        n58 = case shown="\"Minimize\", \"Minimized\"" w210 {
          tunnel: w214 -> [w222 w237 w248 w261 w274]
          tunnel: [w224 w238 w250 w263 w276] -> w213
          tunnel: w211 -> [w223 w235 w249 w262 w275]
          frame "Open", "Standard", Default {
            w217 = T1."Standard" ("State")
            n59 = property class="VI"(reference=w223, error in=w222) -> (reference out=w220:refnum<vi>, error out=w221:errorcluster, "FP.State"=w219:T1)
            n60 = Not Equal?(x=w219, y=w217) -> (x != y?=w218:bool)
            n61 = case shown="True" w218 {
              tunnel: [w228 w230] -> w224
              tunnel: w221 -> [w227 w230]
              tunnel: w220 -> [w226 _]
              tunnel: w217 -> [w225 _]
              frame True {
                n62 = invoke class="VI" method="FP.Open"(reference=w226, error in=w227, "Activate"=TRUE, "State"=w225) -> (error out=w228:errorcluster)  [unwired: 1 in, 4 out]
              }
              frame False {
              }
            }
          }
          frame "Close", "Closed" {
            n63 = property class="VI"(reference=w235, error in=w237) -> (reference out=w234:refnum<vi>, error out=w236:errorcluster, "FP.State"=w232:T1)
            n64 = Not Equal?(x=w232, y=T1."Closed" ("Front Panel Window:State")) -> (x != y?=w231:bool)
            n65 = case shown="True" w231 {
              tunnel: [w239 w242] -> w238
              tunnel: w236 -> [w239 w241]
              tunnel: w234 -> [_ w240]
              frame False {
              }
              frame True {
                n66 = invoke class="VI" method="FP.Close"(reference=w240, error in=w241) -> (error out=w242:errorcluster)  [unwired: 1 in, 2 out]
              }
            }
          }
          frame "Hidden", "Hide" {
            w243 = T1."Hidden" ("State")
            n67 = property class="VI"(reference=w249, error in=w248) -> (reference out=w246:refnum<vi>, error out=w247:errorcluster, "FP.State"=w245:T1)
            n68 = Not Equal?(x=w245, y=w243) -> (x != y?=w244:bool)
            n69 = case shown="True" w244 {
              tunnel: [w254 w255] -> w250
              tunnel: w247 -> [w253 w255]
              tunnel: w246 -> [w252 _]
              tunnel: w243 -> [w251 _]
              frame True {
                n70 = invoke class="VI" method="FP.Open"(reference=w252, error in=w253, "State"=w251) -> (error out=w254:errorcluster)  [unwired: 2 in, 4 out]
              }
              frame False {
              }
            }
          }
          frame "Minimize", "Minimized" {
            w256 = T1."Minimized" ("State")
            n71 = property class="VI"(reference=w262, error in=w261) -> (reference out=w259:refnum<vi>, error out=w260:errorcluster, "FP.State"=w258:T1)
            n72 = Not Equal?(x=w258, y=w256) -> (x != y?=w257:bool)
            n73 = case shown="True" w257 {
              tunnel: [w267 w268] -> w263
              tunnel: w260 -> [w266 w268]
              tunnel: w259 -> [w265 _]
              tunnel: w256 -> [w264 _]
              frame True {
                n74 = invoke class="VI" method="FP.Open"(reference=w265, error in=w266, "State"=w264) -> (error out=w267:errorcluster)  [unwired: 2 in, 4 out]
              }
              frame False {
              }
            }
          }
          frame "Maximize", "Maximized" {
            w269 = T1."Maximized" ("State")
            n75 = property class="VI"(reference=w275, error in=w274) -> (reference out=w272:refnum<vi>, error out=w273:errorcluster, "FP.State"=w271:T1)
            n76 = Not Equal?(x=w271, y=w269) -> (x != y?=w270:bool)
            n77 = case shown="True" w270 {
              tunnel: [w280 w281] -> w276
              tunnel: w273 -> [w279 w281]
              tunnel: w272 -> [w278 _]
              tunnel: w269 -> [w277 _]
              frame True {
                n78 = invoke class="VI" method="FP.Open"(reference=w278, error in=w279, "State"=w277) -> (error out=w280:errorcluster)  [unwired: 2 in, 4 out]
              }
              frame False {
              }
            }
          }
        }
        n79 = call <vilib>:"Add State(s) to Queue__JKI_lib_State_Machine.vi"("State(s) in (\"\")"=w216) -> ("States Out"=w215:string)  [unwired: 14 in]
      }
      frame "---------- Macro ----------" {
        # "Do not put any code in this frame.\n(It is a separator no-op. You can make a copy of this frame to create a new Macro frame)"
        n80 = call <vilib>:"Add State(s) to Queue__JKI_lib_State_Machine.vi"("State(s) in (\"\")"=w286) -> ("States Out"=w285:string)  [unwired: 14 in]
      }
      frame "Macro: Initialize" {
        w288 = "Data: Initialize\nInitialize Core Data\nEvents: Register\nUI: Initialize\nUI: Front Panel State >> Open"  # Data: Initialize Initialize Core Data Events: Register UI: Initialize UI: Front Panel State >> Open
        # "Initialization Macro\n(This is called once, when the VI starts)"
        n81 = call <vilib>:"Add State(s) to Queue__JKI_lib_State_Machine.vi"("State(s) in Front (\"\")"=w288, "State(s) in (\"\")"=w292) -> ("States Out"=w291:string)  [unwired: 13 in]
      }
      frame "Macro: Exit" {
        # "Exit Macro\n(This is called once, when the VI exits)"
        n82 = Unbundle By Name(w300) -> ("Core.Close Panel on Exit?"=w299:bool)
        n83 = Select(t="UI: Front Panel State >> Close", s=w299, f="") -> (s? t:f=w296:string)
        n84 = call <vilib>:"Add State(s) to Queue__JKI_lib_State_Machine.vi"("State(s) in (\"\")"=w296, "State(s) at Back (\"\")"="Data: Cleanup\nEvents: Unregister\nExit") -> ("States Out"=w294:string)  [unwired: 13 in]
        n85 = call <vilib>:"Add State(s) to Queue__JKI_lib_State_Machine.vi"("State(s) in Front (\"\")"=w294, "State(s) in (\"\")"=w303) -> ("States Out"=w302:string)  [unwired: 13 in]
      }
      frame "---------- API ----------" {
        # "Do not put any code in this frame.\n(It is a separator no-op. This category is recommanded to use for external API)"
      }
      frame "API: API1" {
        # "If you need to tell who triggered this state , use this string. If it's this case itself, this string is \"\"."
        # "Deal with the parameter if any"
        # "Connect this to return the response of your API"
        # "Copy/Rename this case for your own API"
      }
      frame "API: API2" {
        # "unpack HexStr  to Variant\nif complex parameter is needed."
        # "Copy/Rename this case for your own API"
        n86 = call <userlib>:"JKISM++ Convert HexStr to Data.vi"("HEX String"=w314) -> ()  [unwired: 8 in, 1 out]
        n87 = disable-structure shown="Enabled" {
          disable-tunnel: [w319 "API2 Response"] -> w313
          frame Disabled {
            # "pack variant to hexstr \nif complex response is needed."
            # "complex Response"
            n88 = call <userlib>:"JKISM++ Convert Data to HexStr.vi"() -> ("HEX String (0-9,A-F)"=w319:string)  [unwired: 9 in]
          }
          frame Enabled {
          }
        }
      }
      frame "---------- DoSth ----------" {
        # "Template Separator\n(You can make a copy of, or modify, this frame)"
        n89 = call <vilib>:"Add State(s) to Queue__JKI_lib_State_Machine.vi"("State(s) in (\"\")"=w325) -> ("States Out"=w324:string)  [unwired: 14 in]
      }
      frame "DoSth: DoA" {
        # "Your code here.\n(You can make a copy of, or modify, this frame)"
        n90 = call <vilib>:"Add State(s) to Queue__JKI_lib_State_Machine.vi"("State(s) in (\"\")"=w331) -> ("States Out"=w330:string)  [unwired: 14 in]
      }
      frame "DoSth: DoB" {
        # "Your code here.\n(You can make a copy of, or modify, this frame)"
        n91 = call <vilib>:"Add State(s) to Queue__JKI_lib_State_Machine.vi"("State(s) in (\"\")"=w337) -> ("States Out"=w336:string)  [unwired: 14 in]
      }
    }
  }
